vi "Get Object from Class Path.vi"(0 "LabVIEW Class Path":path, 5 "Options":u32, 11 "error in (no error)":errorcluster) -> (4 "Object":refnum<class>, 15 "error out":errorcluster)   [LabVIEW 2016, in "SLL Class.lvlib"]
doc: "This method is an optimized version of using the default \"Get LabVIEW Class Default Value\" to get the class object from the class path. \n\nIt stores the class object in a Variant lookup table, so that the next time when the same class object is required, it would get it from the Variant lookup table, which is faster."
uses:
  SLL Class.lvlib
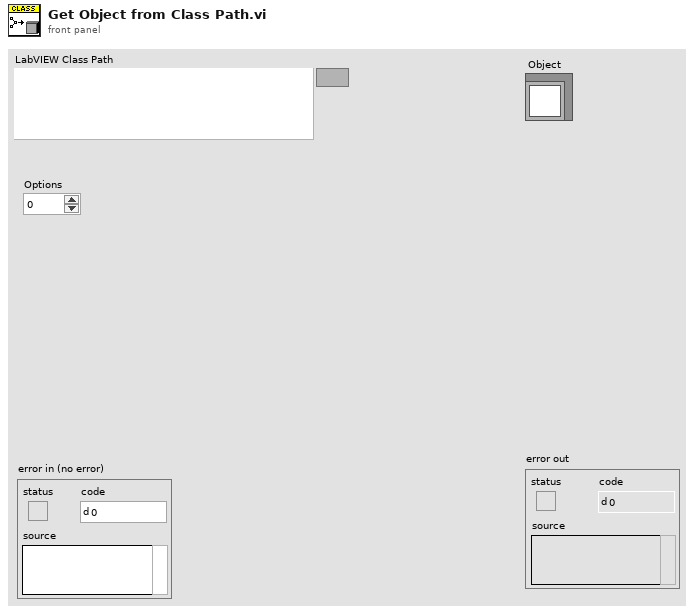
[diagram p1: front panel]
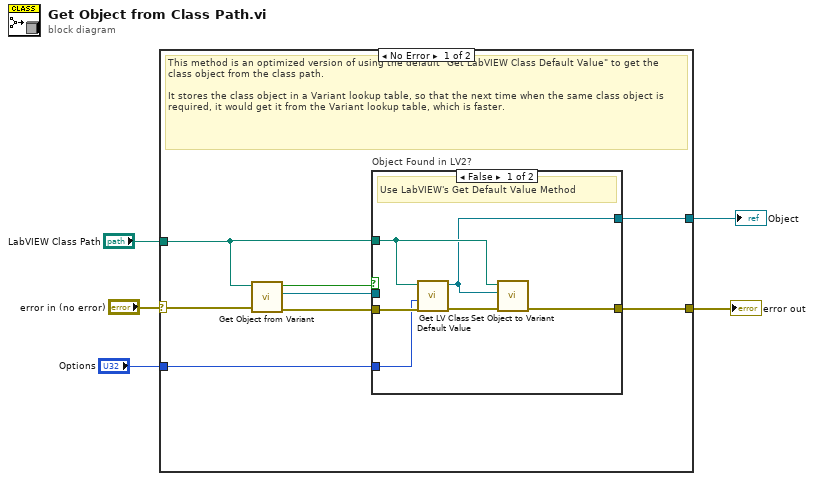
[diagram p0: block diagram]
diagram:
  n1 = case shown="No Error" "error in (no error)" {
    selector: "error in (no error)" -> [w11 w22]
    tunnel: [w13 _] -> w5
    tunnel: [w12 w22] -> w4
    tunnel: "LabVIEW Class Path" -> [w7 _]
    tunnel: "Options" -> [w6 _]
    frame No Error {
      # "This method is an optimized version of using the default \"Get LabVIEW Class Default Value\" to get the class object from the class path. \n\nIt stores the class object in a Variant lookup table, so that the next time when the same class object is required, it would get it from the Variant lookup table, which is faster."
      n2 = call "Get Object from Variant.vi"("error in (no error)"=w11, "LabVIEW Class Path"=w7) -> ("error out"=w8:errorcluster, "Object"=w9:refnum<class>, "Found?"=w10:bool)  [unwired: 7 in]
      n3 = case "Object Found in LV2?" shown="False" w10 {
        tunnel: [w15 w21] -> w13
        tunnel: [w17 w20] -> w12
        tunnel: w9 -> [_ w21]
        tunnel: w8 -> [w19 w20]
        tunnel: w7 -> [w16 _]
        tunnel: w6 -> [w14 _]
        frame False {
          # "Use LabVIEW's Get Default Value Method"
          n4 = call <vilib>:"Get LV Class Default Value.vi"("error in (no error)"=w19, "options"=w14, "class path"=w16) -> ("error out"=w18:errorcluster, "object"=w15:refnum<class>)  [unwired: 7 in]
          n5 = call "Set Object to Variant.vi"("error in (no error)"=w18, "Object"=w15, "LabVIEW Class Path"=w16) -> ("error out"=w17:errorcluster)  [unwired: 8 in]
        }
        frame True {
          # "Use the Object from the Variant LUT"
        }
      }
    }
    frame Error {
    }
  }
  "Object" <- w5
  "error out" <- w4
